vi "flattenTemperatureAbsToXML_Scalar.vi"(8 "error in (no error)":errorcluster, 9 "temperatureAbsUnitInXML":T1, 10 "temperatureAbsAgain":variant, 11 "temperatureAbs":dbl[unit]=273.15) -> (0 "error out":errorcluster, 3 "xmlString":string)   [LabVIEW 2016, in "UnitsAndXML.lvlib"]
uses:
  <userlib>/Common/UnitsAndXML/UnitsAndXML.lvlib
  <userlib>/Common/UnitsAndXML/FlattenItemWithUnitToXML/FlattenTemperatureAbsToXML/TemperatureAbsUnit.ctl
  <vilib>/Utility/VariantDataType/VariantType.lvlib
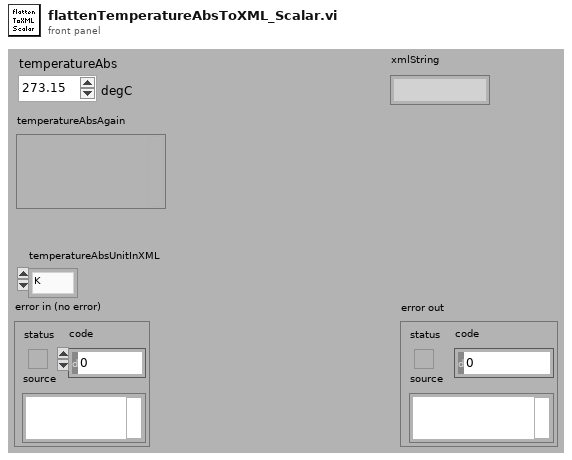
[diagram p1: front panel]
types:
  T1 = typedef "UnitsAndXML.lvlib/TemperatureAbsUnit.ctl" = enum16{"K", "degC", "degF"}
  T2 = typedef "VariantType.lvlib/Type.ctl" = enum8{"Invalid Type", "Void", "I8", "I16", "I32", "I64", "U8", "U16", "U32", "U64", "Single Float", "Double Float", "Extended Float", "Single Complex", "Double Complex", "Extended Complex", "Enum U8", "Enum U16", "Enum U32", "Enum U64", "Single Float With Unit", "Double Float With Unit", "Extended Float With Unit", "Single Complex with Unit", "Double Complex with Unit", "Extended Complex with Unit", "Boolean", "String", "Path", "Picture", "Tag", "Array", "Cluster", "Variant", "LV Variant", "Waveform", "Timestamp", "Digital Waveform", "Digital Data", "ExpressData", "Refnum", "External Data", "VI", "Poly VI", "LabVIEW Class Instance", "Fixed Point"}
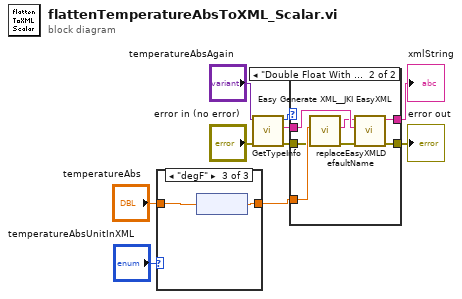
[diagram p0: block diagram]
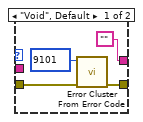
[diagram p2: hidden frame]
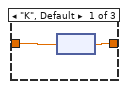
[diagram p3: hidden frame]
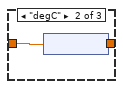
[diagram p4: hidden frame]
diagram:
  n1 = case shown="\"degF\"" "temperatureAbsUnitInXML" {
    tunnel: "temperatureAbs" -> [w12 w14 w16]
    tunnel: [w11 w13 w15] -> w10
    frame "K", Default {
      n2 = node(w12) -> (w11:dbl)
    }
    frame "degC" {
      n3 = node(w14) -> (w13:dbl)
    }
    frame "degF" {
      n4 = node(w16) -> (w15:dbl)
    }
  }
  n5 = call <vilib>:"GetTypeInfo.vi"("error in (no error)"="error in (no error)", "Variant"="temperatureAbsAgain") -> ("error out"=w2:errorcluster, "Name"=w1:string, "Type Enum"=w3:T2)  [unwired: 5 in, 2 out]
  n6 = case shown="\"Double Float With Unit\"" w3 {
    tunnel: w10 -> [_ w27]
    tunnel: ["" w26] -> w7
    tunnel: [w19 w25] -> w6
    tunnel: w2 -> [w17 w22]
    tunnel: w1 -> [_ w24]
    frame "Void", Default {
      n7 = call <vilib>:"Error Cluster From Error Code.vi"("error in (no error)"=w17, "error code (0)"=9101) -> ("error out"=w19:errorcluster)  [unwired: 7 in]
    }
    frame "Double Float With Unit" {
      n8 = call <vilib>:"Easy Generate XML__JKI EasyXML.vi"("error in (no error)"=w22, "LabVIEW Data"=w27) -> ("error out"=w21:errorcluster, "XML String"=w23:string)  [unwired: 8 in]
      n9 = call <userlib>:"replaceEasyXMLDefaultName.vi"("error in"=w21, "desiredName"=w24, "easyXMLStringWithDefaultNames"=w23) -> ("error out"=w25:errorcluster, "xmlString"=w26:string)  [unwired: 7 in]
    }
  }
  "xmlString" <- w7
  "error out" <- w6
